vi "Create References.vi"(8 "error in":errorcluster, 9 "BD Win.Origin":T1, 11 "Controls[]":refnum<vi>[](array[refnum])) -> (0 "error out":errorcluster, 1 "References[]":refnum<vi>[](array[refnum]), 2 "Vertical Center":i32, 3 "Right":i16)   [LabVIEW 2012, in "Build Cluster of References__RCF.lvlib"]
doc: "Creates a reference for each control in the Controls[] array, moves its label to the left and compresses the references vertically."
uses:
  Build Cluster of References__RCF.lvlib
  <vilib>/Utility/miscctls.llb/LVPointTypeDef.ctl
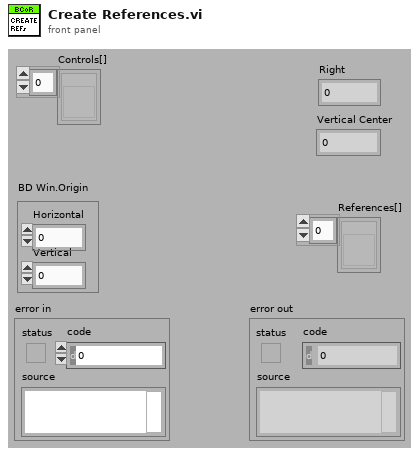
[diagram p1: front panel]
types:
  T1 = typedef "LVPointTypeDef.ctl" = cluster{"Horizontal":i16, "Vertical":i16}
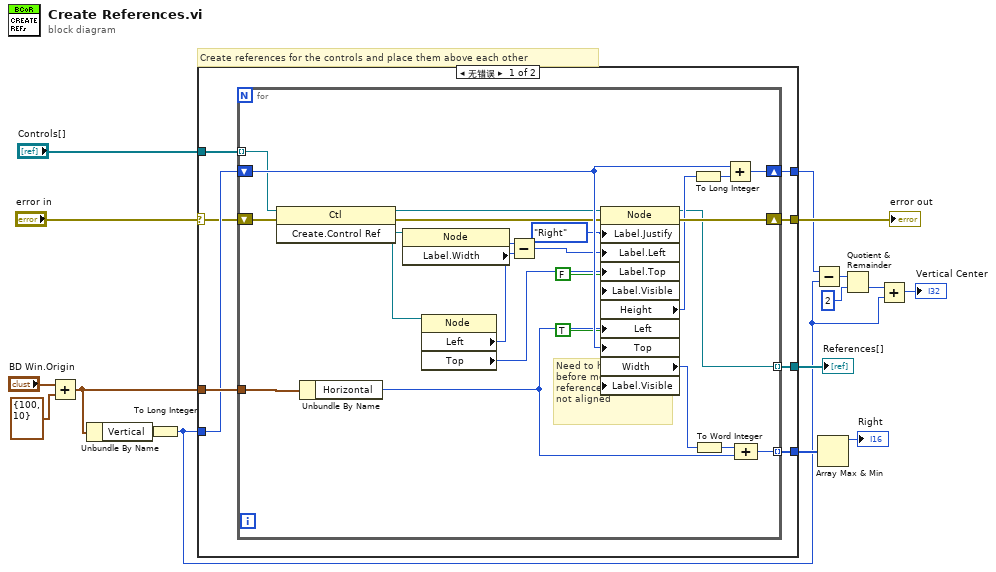
[diagram p0: block diagram]
diagram:
  # "Create references for the controls and place them above each other"
  n1 = Add(x="BD Win.Origin", y=T1 {"Horizontal"=100, "Vertical"=10} ("BD Win.Origin")) -> (x+y=w12:T1)
  n2 = Unbundle By Name(w12) -> ("Vertical"=w11:i16)
  n3 = To Long Integer(number=w11) -> (32bit integer=w2:i32)
  n4 = case shown="无错误" "error in" {
    selector: "error in" -> [w20 w47]
    tunnel: [w17 _] -> w16
    tunnel: [w19 w47] -> w15
    tunnel: [w24 _] -> w9
    tunnel: "Controls[]" -> [w23 _]
    tunnel: w12 -> [w22 _]
    tunnel: w2 -> [w21 _]
    tunnel: [w18 _] -> w4
    frame No Error {
      n5 = for {
        tunnel: w23 -> [w41] mode=indexing
        shift-right: [w45] -> w24
        shift-left: w21 -> [w46]
        tunnel: w22 -> [w44]
        shift-right: [w43] -> w19
        shift-left: w20 -> [w40]
        tunnel: [w42] -> w18 mode=indexing
        tunnel: [w25] -> w17 mode=indexing
        # "Need to hide the label before moving the references, or they're not aligned"
        n6 = invoke class="Ctl" method="Create.Control Ref"(reference=w41, error in=w40) -> (error out=w32:errorcluster, "Create Control Ref"=w38:refnum<vi>)  [unwired: 1 in, 1 out]
        n7 = Unbundle By Name(w44) -> ("Horizontal"=w29:i16)
        n8 = property class="Node"(reference=w38) -> ("Label.Width"=w36:u32)  [unwired: 1 in, 2 out]
        n9 = property class="Node"(reference=w38) -> ("Left"=w35:i32, "Top"=w37:i32)  [unwired: 1 in, 2 out]
        n10 = Subtract(x=w35, y=w36) -> (x-y=w34:u32)
        n11 = property class="Node"(reference=w38, error in=w32, "Label.Justify"=enum16{"Left", "Center", "Right"}."Right" ("Label.Justification"), "Label.Left"=w34, "Label.Top"=w37, "Label.Visible"=FALSE, "Left"=w29, "Top"=w46, "Label.Visible"=TRUE) -> (reference out=w25:refnum<vi>, error out=w43:errorcluster, "Height"=w33:u32, "Width"=w27:u32)
        n12 = To Long Integer(number=w33) -> (32bit integer=w26:i32)
        n13 = To Word Integer(number=w27) -> (16bit integer=w28:i16)
        n14 = Add(x=w46, y=w26) -> (x+y=w45:i32)
        n15 = Compound Arithmetic op=ADD(w28, w29) -> (w42:i16)
      }
    }
    frame Error {
    }
  }
  "References[]" <- w16
  "error out" <- w15
  n16 = Subtract(x=w9, y=w2) -> (x-y=w7:i32)
  n17 = Array Max & Min(array=w4) -> (max value=→"Right":i16)  [unwired: 3 out]
  n18 = Quotient & Remainder(x=w7, y=2) -> (floor(x/y)=w6:i32)  [unwired: 1 out]
  n19 = Add(x=w6, y=w2) -> (x+y=→"Vertical Center":i32)
